vi "Actor Core.vi"(8 "error in":errorcluster, 11 "Pulse Controller in":refnum<class "Pulse Controller.lvclass">) -> (0 "error out":errorcluster, 3 "Actor out":refnum<class "Actor.lvclass">)   [LabVIEW 2018, in "Pulse Controller.lvclass"]
doc: "(<B>Filename</B>: Actor Framework.lvlib:Actor.lvclass:Actor Core.vi)\n\nReceives messages to the actor, reacts to them, and initiates any error handling that may shut the actor down.\n\nDescendant classes may override this VI to append parallel tasks for the actor to complete while it handles messages. Overrides use the Call Parent Method node."
uses:
  Pulse Controller.lvclass
  C:/github/2018/LabActor/Template Module/Template Module.lvclass
  C:/github/2018/LabActor/Controllers/Process Controller/Process Controller.lvclass
  C:/Program Files/National Instruments/LabVIEW 2018/vi.lib/ActorFramework/Actor/Actor.lvclass
  <vilib>/ActorFramework/Actor/Actor.lvclass
  Pulse Controller Configuration.ctl
  Template Module/Template Module.lvclass/Template Module.ctl
  Process Controller/Process Controller.lvclass/Process Controller.ctl
  <vilib>/ActorFramework/Actor/Actor.lvclass/Actor.ctl
  <vilib>/ActorFramework/Message Enqueuer/Message Enqueuer.lvclass/Message Enqueuer.ctl
  Template Module/Read stop event.vi
  Process Controller/Write Log Init Response.vi
  <vilib>/ActorFramework/Message Enqueuer/Init from Existing Queue.vi
  <vilib>/ActorFramework/Message Enqueuer/Enqueue.vi
  Worker Messages/Trigger Msg/Trigger Msg.lvclass
  C:/Program Files/National Instruments/LabVIEW 2018/vi.lib/ActorFramework/Message/Message.lvclass
  <vilib>/ActorFramework/Message Priority Queue/Priority Enqueue.vi
  Process Controller/Process Controller.lvclass
  <vilib>/ActorFramework/Message Enqueuer/Message Enqueuer.lvclass
panel:
  in  "Trigger":bool
  in  "Configuration":T1={"Pre-trigger duration"=-1.0, "Post-trigger duration"=-1.0, "Open plot after pulse"=TRUE} {"Pre-trigger duration" format="%#_6p"; "Post-trigger duration" format="%#_6p"}
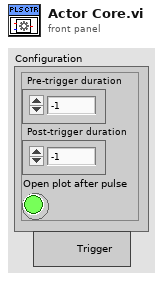
[diagram p1: front panel]
types:
  T1 = typedef "Pulse Controller Configuration.ctl" = cluster{"Pre-trigger duration":dbl, "Post-trigger duration":dbl, "Open plot after pulse":bool}
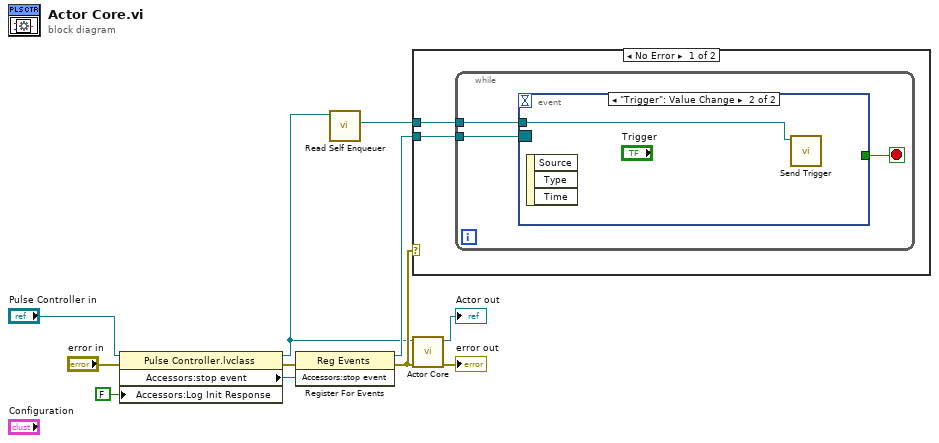
[diagram p0: block diagram]
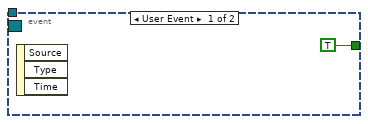
[diagram p2: hidden frame]
diagram:
  n1 = property class="Pulse Controller.lvclass"(reference="Pulse Controller in", error in="error in", "Accessors:Log Init Response"=FALSE ("Log Init Response")) -> (reference out=w2:refnum<class "Pulse Controller.lvclass">, error out=w9:errorcluster, "Accessors:stop event"=w8:refnum<user-event>)
  n2 = register-events(error in=w9, w8) -> (reference out=w6:refnum<event-registration>, error out=w3:errorcluster)  [unwired: 1 in]
  n3 = call <vilib>:"Read Self Enqueuer.vi"("Actor"=w2) -> ("Self Enqueuer"=w7:refnum<class "Message Enqueuer.lvclass">)  [unwired: 10 in]
  n4 = case shown="No Error" w3 {
    tunnel: w6 -> [w13 _]
    tunnel: w7 -> [w12 _]
    frame No Error {
      n5 = while {
        tunnel: w13 -> [w16]
        tunnel: w12 -> [w14]
        stop <- w15 stop-if-true
        n6 = event shown="[1] \"Trigger\": Value Change" {
          selector: w16 -> [_ _]
          dyn-events: _ -> [_ _]
          timeout: _ -> [_ _]
          tunnel: [TRUE _] -> w15
          tunnel: w14 -> [_ w18]
          event User Event {
            n7 = event-data() -> ()  [unwired: 1 in, 3 out]
          }
          event "Trigger": Value Change {
            n8 = event-data() -> ()  [unwired: 1 in, 3 out]
            n9 = call "Send Trigger.vi"("Message Enqueuer"=w18) -> ()  [unwired: 9 in, 2 out]
          }
        }
      }
    }
    frame Error {
    }
  }
  n10 = call-parent "Actor Core.vi"("error in"=w3, "Measure Object in"=w2) -> ("error out"=→"error out":errorcluster, "Actor out"=→"Actor out":refnum<class "Actor.lvclass">)  [unwired: 8 in]
